vi "RenameClassSpecific.vi"(0 "ClassWriterGOOP300.lvclass":refnum<class "ClassWriterGOOP400.lvclass">, 1 "ClassRef":refnum<vi>, 2 "NewClassPath":path, 5 "error in":errorcluster) -> (14 "ClassWriterGOOP300.lvclass 2":refnum<class "ClassWriterGOOP400.lvclass">, 19 "error out":errorcluster)   [LabVIEW 2020, in "ClassWriterGOOP400.lvclass"]
uses:
  <resource>/Framework/Providers/Open_GDS/ClassProviders/Provider_EndevoGOOP400/ClassWriterGOOP400_class/ClassWriterGOOP400.lvclass
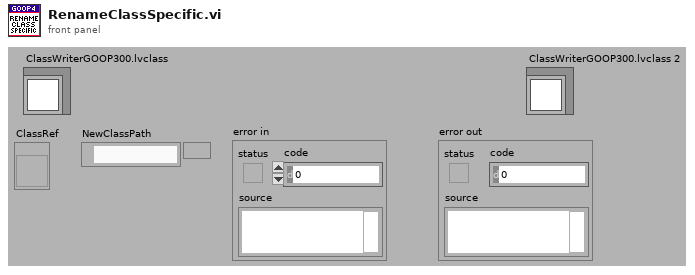
[diagram p1: front panel]
types:
  T1 = typedef "imagedata.ctl" = cluster{"image type":i32, "image depth":i32, "image":u8[], "mask":u8[], "colors":u32[], "Rectangle":cluster{"left":i16, "top":i16, "right":i16, "bottom":i16}}
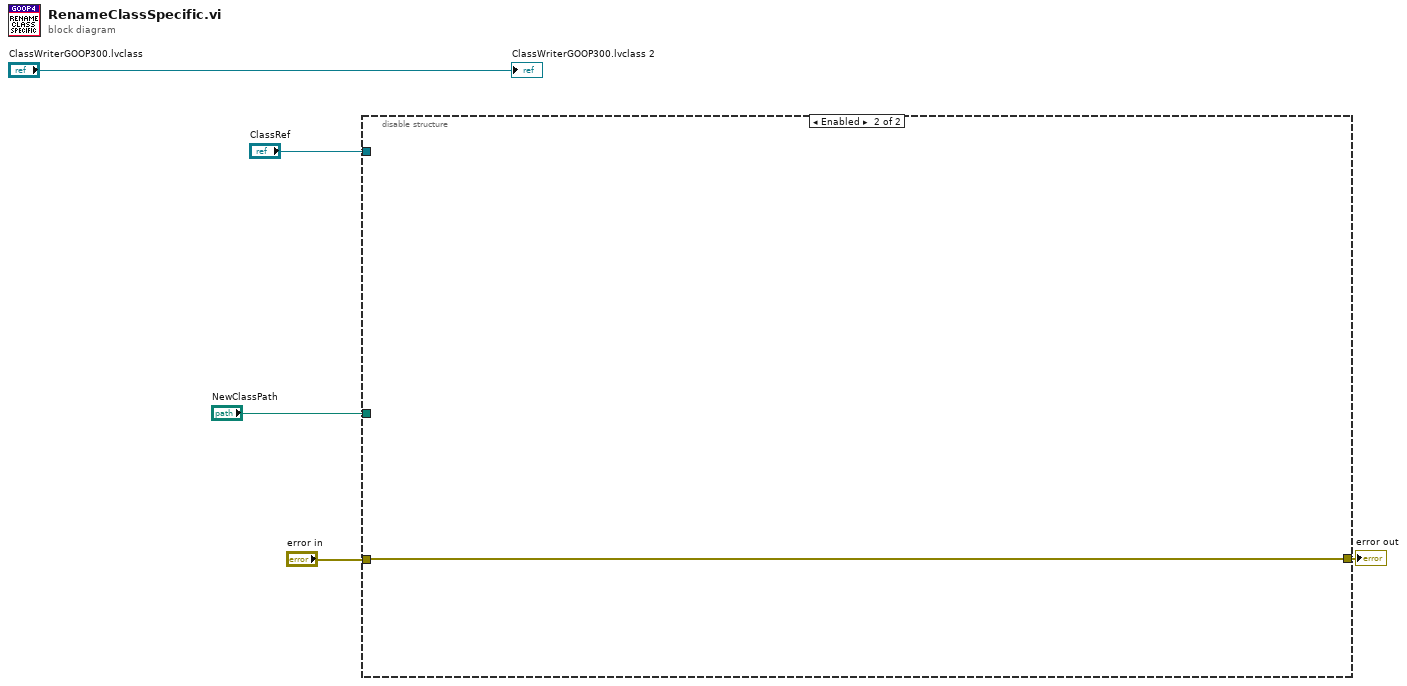
[diagram p0: block diagram]
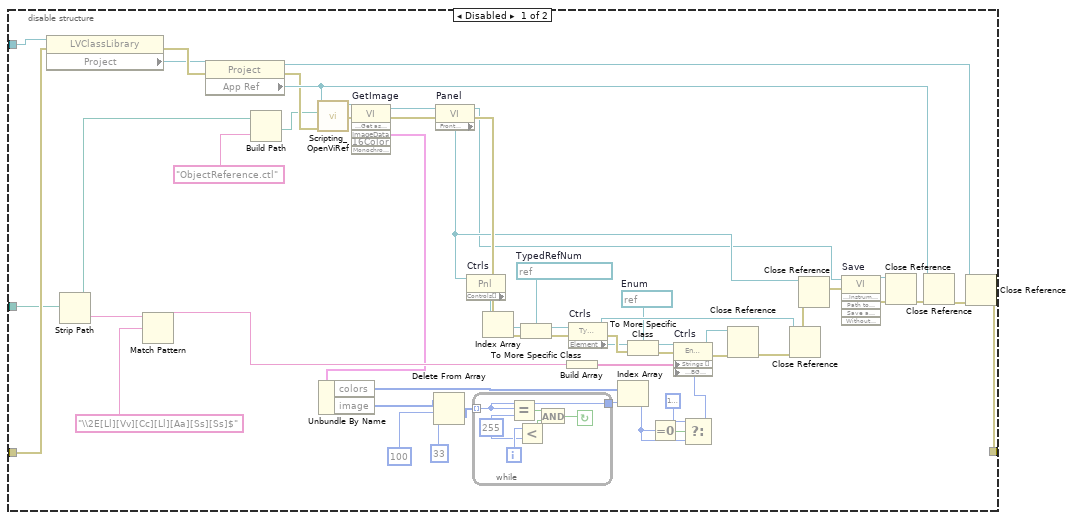
[diagram p2: hidden frame]
diagram:
  n1 = disable-structure shown="Enabled" {
    disable-tunnel: [w58 w66] -> w5
    disable-tunnel: "error in" -> [w52 w66]
    disable-tunnel: "ClassRef" -> [w50 _]
    disable-tunnel: "NewClassPath" -> [w48 _]
    frame Disabled {
      w12 = refnum<vi> refnum  # Enum
      w9 = refnum<vi> refnum  # TypedRefNum
      n2 = property class="LVClassLibrary"(reference=w50, error in=w52) -> (error out=w53:errorcluster, "Project"=w51:refnum<vi>)  [unwired: 1 out]
      n3 = Strip Path(path=w48) -> (stripped path=w49:path, name=w55:string)
      n4 = Match Pattern(string=w55, regular expression="\\2E[Ll][Vv][Cc][Ll][Aa][Ss][Ss]$" ("string")) -> (before substring=w56:string)  [unwired: 1 in, 3 out]
      n5 = property class="Project"(reference=w51, error in=w53) -> (reference out=w59:refnum<vi>, error out=w41:errorcluster, "App Ref"=w47:refnum<vi>)
      n6 = Build Path(base path=w49, name or relative path="ObjectReference.ctl") -> (appended path=w40:path)
      n7 = call <resource>:"Scripting_OpenViRef.vi"("error in"=w41, "ViPath/ViName/Viref"=w40, "AppRef"=w47) -> ("error out"=w28:errorcluster, "vi reference"=w27:refnum<vi>)  [unwired: 6 in, 1 out]
      n8 = invoke on="GetImage" class="VI" method="VI Icon.Get as Image Data"(reference=w27, error in=w28) -> (reference out=w29:refnum<vi>, error out=w30:errorcluster, "ImageData"=w31:T1)  [unwired: 4 in, 3 out]
      n9 = Unbundle By Name(w31) -> ("colors"=w34:u32[], "image"=w32:u8[])
      n10 = Delete From Array(array=w32, length=100, index=33) -> (deleted portion=w42:u8[])  [unwired: 1 out]
      n11 = property on="Panel" class="VI"(reference=w29, error in=w30) -> (reference out=w23:refnum<vi>, error out=w45:errorcluster, "Front Panel"=w44:refnum<vi>)
      n12 = property on="Ctrls" class="Pnl"(reference=w44, error in=w45) -> ("Controls[]"=w7:refnum<vi>[])  [unwired: 2 out]
      n13 = while {
        tunnel: w42 -> [w60] mode=indexing
        tunnel: [w60] -> w43
        i -> [w64]
        stop <- w61 continue-if-true
        w63 = 255
        n14 = Equal?(x=w60, y=w63) -> (x = y?=w65:bool)
        n15 = Less?(x=w64, y=w63) -> (x < y?=w62:bool)
        n16 = And(x=w65, y=w62) -> (x .and. y?=w61:bool)
      }
      n17 = Index Array(array=w7) -> (element=w8:refnum<vi>)  [unwired: 1 in]
      n18 = To More Specific Class(target class=w9, reference=w8, error in=w45) -> (specific class reference=w10:refnum<vi>, error out=w15:errorcluster)
      n19 = Build Array(w56) -> (w14:string[])
      n20 = property on="Ctrls" class="TypRef"(reference=w10, error in=w15) -> (reference out=w21:refnum<vi>, error out=w16:errorcluster, "Element"=w11:refnum<vi>)
      n21 = Index Array(array=w34, index=w43) -> (element=w37:u32)
      n22 = To More Specific Class(target class=w12, reference=w11, error in=w16) -> (specific class reference=w13:refnum<vi>, error out=w17:errorcluster)
      n23 = Equal To 0?(x=w37) -> (x = 0?=w36:bool)
      n24 = Select(t=u32 16777216, s=w36, f=w37) -> (s? t:f=w38:u32)
      n25 = property on="Ctrls" class="Enum"(reference=w13, error in=w17, "Strings []"=w14, "Named Numeric Colors:BG Color"=w38) -> (reference out=w18:refnum<vi>, error out=w19:errorcluster)
      n26 = Close Reference(reference=w18, error in (no error)=w19) -> (error out=w20:errorcluster)
      n27 = Close Reference(reference=w21, error in (no error)=w20) -> (error out=w22:errorcluster)
      n28 = Close Reference(reference=w44, error in (no error)=w22) -> (error out=w24:errorcluster)
      n29 = invoke on="Save" class="VI" method="Save.Instrument"(reference=w23, error in=w24) -> (reference out=w25:refnum<vi>, error out=w26:errorcluster)  [unwired: 4 in, 4 out]
      n30 = Close Reference(reference=w25, error in (no error)=w26) -> (error out=w46:errorcluster)
      n31 = Close Reference(reference=w47, error in (no error)=w46) -> (error out=w57:errorcluster)
      n32 = Close Reference(reference=w59, error in (no error)=w57) -> (error out=w58:errorcluster)
    }
    frame Enabled {
    }
  }
  "error out" <- w5
  "ClassWriterGOOP300.lvclass 2" <- "ClassWriterGOOP300.lvclass"
